vi "SeCrTs-DO_Scale_Config.vi"(8 "error in (no error)":errorcluster, 10 "DO config":T1(array[cluster]), 11 "Refnum in":refnum<k21>) -> (0 "error out":errorcluster, 1 "Array 2":string[](array[string]), 2 "Array":bool[](array[boolean]), 3 "Refnum out":refnum<k21>)   [LabVIEW 2022 SP3]
uses:
  <vilib>/DAQmx/create/channels.llb/DAQmx Create Channel (DO-Digital Output).vi
  <resource>/objmgr/daqmx.rc
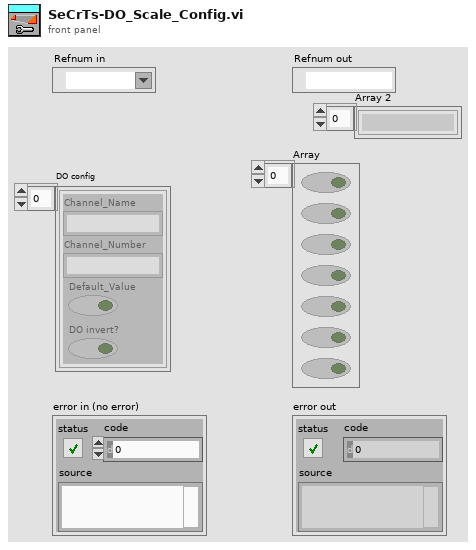
[diagram p1: front panel]
types:
  T1 = cluster{"Channel_Name":string, "Channel_Number":string, "Default_Value":bool, "DO invert?":bool}[]
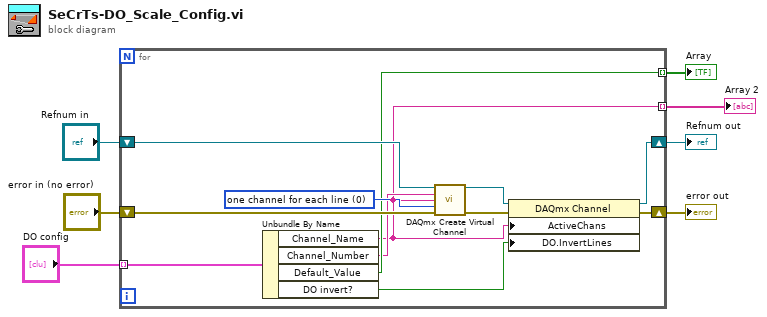
[diagram p0: block diagram]
diagram:
  n1 = for {
    tunnel: "DO config" -> [w19] mode=indexing
    shift-right: [w13] -> w3
    shift-left: "Refnum in" -> [w18]
    shift-right: [w12] -> w4
    shift-left: "error in (no error)" -> [w17]
    tunnel: [w15] -> w5 mode=indexing
    tunnel: [w8] -> w1 mode=indexing
    w16 = 0 items=["one channel for each line", "one channel for all lines"] ("line grouping")
    n2 = Unbundle By Name(w19) -> ("Channel_Name"=w8:string, "Channel_Number"=w9:string, "Default_Value"=w15:bool, "DO invert?"=w10:bool)
    n3 = call-poly <vilib>:"DAQmx Create Virtual Channel.vi"("task in"=w18, "lines"=w9, "name to assign"=w8, "line grouping"=w16, "error in"=w17) -> ("task out"=w14:refnum<k21>, "error out"=w11:errorcluster)  [unwired: 9 in]
    n4 = property on="Property Node" class="DAQmx Channel"(reference=w14, error in=w11, "ActiveChans"=w8, "DO.InvertLines"=w10) -> (reference out=w13:refnum<k21>, error out=w12:errorcluster)
  }
  "Array" <- w5
  "error out" <- w4
  "Refnum out" <- w3
  "Array 2" <- w1
